vi "TestAll.vi"() -> ()   [LabVIEW 2010]
uses:
  Create Dataset 3D Integer.vi
  Append To Dataset 3D Integer.vi
panel:
  in  "Dataset name":string="Bar"
  in  "Group name":string="Foo"
  out "dataset_id":i32=83886080
  out "file_id":i32=16777217
  out "group_id":i32=33554433
  in  "File name":string="C:\\test"
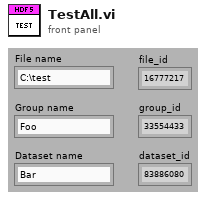
[diagram p1: front panel]
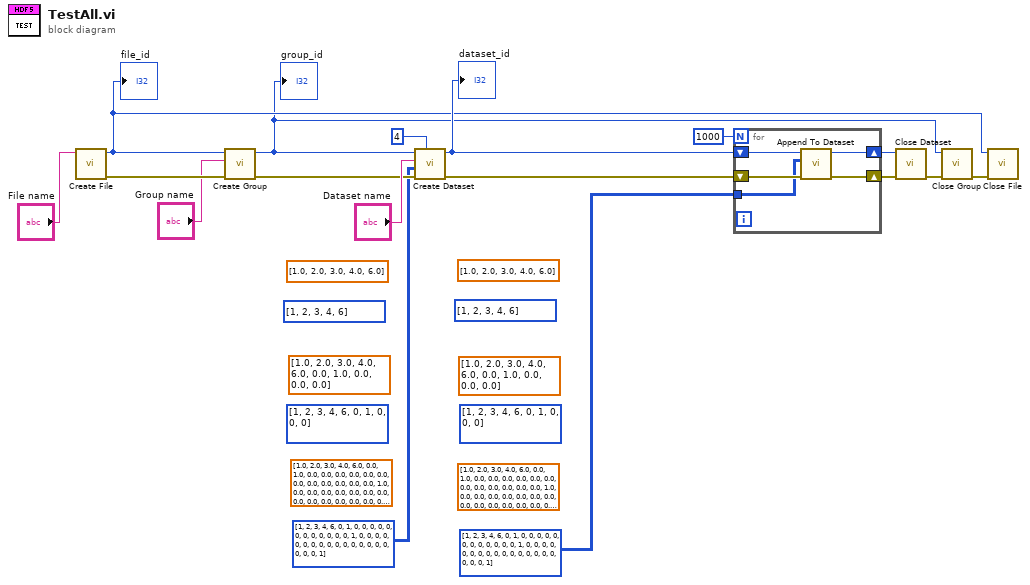
[diagram p0: block diagram]
diagram:
  (unwired) dbl[][][] [[[1.0, 2.0, 3.0, 4.0, 6.0], [0.0, 1.0, 0.0, 0.0, 0.0]], [[0.0, 0.0, 0.0, 0.0, 0.0], [0.0, 0.0, 0.0, 0.0, 1.0]], [[0.0, 0.0, 0.0, 0.0, 0.0], [0.0, 0.0, 0.0, 0.0, 0.0]], [[0.0, 0.0, 0.0, 0.0, 0.0], [0.0, 0.0, 0.0, 0.0, 1.0]]]
  (unwired) dbl[][][] [[[1.0, 2.0, 3.0, 4.0, 6.0], [0.0, 1.0, 0.0, 0.0, 0.0]], [[0.0, 0.0, 0.0, 0.0, 0.0], [0.0, 0.0, 0.0, 0.0, 1.0]], [[0.0, 0.0, 0.0, 0.0, 0.0], [0.0, 0.0, 0.0, 0.0, 0.0]], [[0.0, 0.0, 0.0, 0.0, 0.0], [0.0, 0.0, 0.0, 0.0, 1.0]]]
  (unwired) i32[] [1, 2, 3, 4, 6]
  (unwired) dbl[] [1.0, 2.0, 3.0, 4.0, 6.0]
  (unwired) i32[] [1, 2, 3, 4, 6]
  (unwired) dbl[] [1.0, 2.0, 3.0, 4.0, 6.0]
  (unwired) i32[][] [[1, 2, 3, 4, 6], [0, 1, 0, 0, 0]]
  (unwired) i32[][] [[1, 2, 3, 4, 6], [0, 1, 0, 0, 0]]
  (unwired) dbl[][] [[1.0, 2.0, 3.0, 4.0, 6.0], [0.0, 1.0, 0.0, 0.0, 0.0]]
  (unwired) dbl[][] [[1.0, 2.0, 3.0, 4.0, 6.0], [0.0, 1.0, 0.0, 0.0, 0.0]]
  n1 = call "Create File.vi"("File name"="File name") -> ("Error out"=w10:errorcluster, "file_id"=w3:i32)  [unwired: 7 in]
  "file_id" <- w3
  n2 = call "Create Group.vi"("error in (no error)"=w10, "Group name"="Group name", "Location id in"=w3) -> ("error out"=w11:errorcluster, "Group id"=w2:i32)  [unwired: 7 in]
  "group_id" <- w2
  n3 = call-poly "Create Dataset.vi"("Chunk size"=u64 4 ("Size of dimension 1"), "error in (no error)"=w11, "Datatype"=i32[][][] [[[1, 2, 3, 4, 6], [0, 1, 0, 0, 0]], [[0, 0, 0, 0, 0], [0, 0, 0, 0, 1]], [[0, 0, 0, 0, 0], [0, 0, 0, 0, 0]], [[0, 0, 0, 0, 0], [0, 0, 0, 0, 1]]], "Dataset name"="Dataset name", "loc_id"=w2) -> ("error out"=w14:errorcluster, "Dataset id"=w12:i32)  [unwired: 5 in]
  "dataset_id" <- w12
  n4 = for {
    N: 1000 -> [_]
    shift-right: [w20] -> w6
    shift-left: w14 -> [w19]
    shift-right: [w21] -> w1
    shift-left: w12 -> [w22]
    tunnel: i32[][][] [[[1, 2, 3, 4, 6], [0, 1, 0, 0, 0]], [[0, 0, 0, 0, 0], [0, 0, 0, 0, 1]], [[0, 0, 0, 0, 0], [0, 0, 0, 0, 0]], [[0, 0, 0, 0, 0], [0, 0, 0, 0, 1]]] -> [w18]
    n5 = call-poly "Append To Dataset.vi"("error in (no error)"=w19, "data"=w18, "dataset_id"=w22) -> ("error out"=w20:errorcluster, "Dataset id out"=w21:i32)  [unwired: 7 in]
  }
  n6 = call "Close Dataset.vi"("error in (no error)"=w6, "dataset_id"=w1) -> ("error out"=w5:errorcluster)  [unwired: 9 in]
  n7 = call "Close Group.vi"("error in (no error)"=w5, "group_id"=w2) -> ("error out"=w4:errorcluster)  [unwired: 9 in]
  n8 = call "Close File.vi"("error in (no error)"=w4, "file_id"=w3) -> ()  [unwired: 9 in, 1 out]
